vi "Quadratic_Solver.vi"() -> ()   [LabVIEW 2022 SP3]
panel:
  out "Root 2":dbl format="%#_13g"
  out "Root 1":dbl format="%#_13g"
  in  "C":dbl
  in  "B":dbl
  in  "A":dbl
  # "Quadratic_Solver:\nFor a given quadratic equation, \nenter the coefficient values of \nA, B, and C to find the roots."
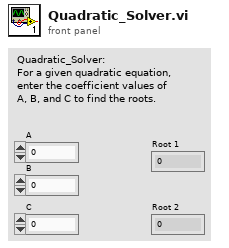
[diagram p1: front panel]
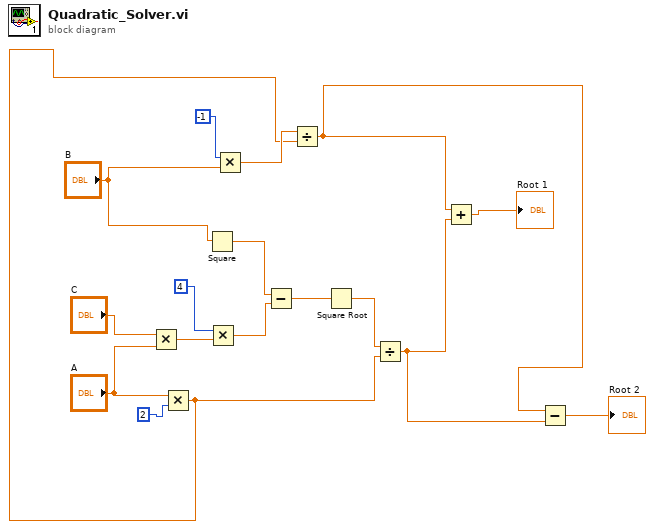
[diagram p0: block diagram]
diagram:
  n1 = Multiply(x="C", y="A") -> (x*y=w16:dbl)
  n2 = Multiply(x="A", y=2) -> (x*y=w6:dbl)
  n3 = Square(x="B") -> (x^2=w15:dbl)
  n4 = Multiply(x=4, y=w16) -> (x*y=w14:dbl)
  n5 = Multiply(x=-1, y="B") -> (x*y=w7:dbl)
  n6 = Subtract(x=w15, y=w14) -> (x-y=w13:dbl)
  n7 = Divide(x=w7, y=w6) -> (x/y=w3:dbl)
  n8 = Square Root(x=w13) -> (sqrt(x)=w5:dbl)
  n9 = Divide(x=w5, y=w6) -> (x/y=w2:dbl)
  n10 = Add(x=w3, y=w2) -> (x+y=→"Root 1":dbl)
  n11 = Subtract(x=w3, y=w2) -> (x-y=→"Root 2":dbl)
